vi "LightOffCommand_Create.vi"(8 "error in (no error)":errorcluster, 10 "Light":refnum<class "Light.lvclass">, 11 "reference in":refnum<class "LightOffCommand.lvclass">) -> (0 "error out":errorcluster, 3 "reference out":refnum<class "LightOffCommand.lvclass">)   [LabVIEW 2020, in "LightOffCommand.lvclass"]
uses:
  LightOffCommand.lvclass
  C:/Projects/OpenGDS_DesignPatterns/Command1/Command_class/Command.lvclass
  Light_class/Light.lvclass
  Command_class/Command.lvclass
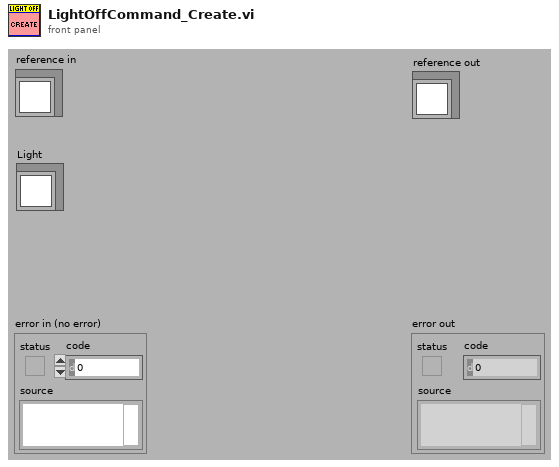
[diagram p1: front panel]
types:
  T1 = typedef "LightOffCommand.lvclass/ObjectAttributes.ctl" = cluster{"Light":refnum<class "Light.lvclass">}
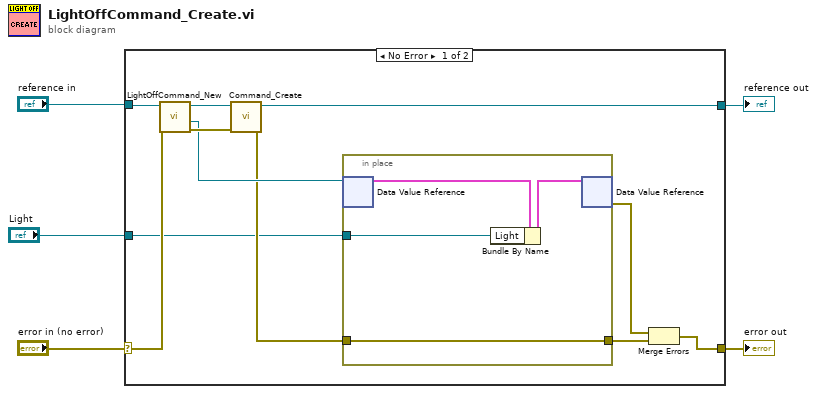
[diagram p0: block diagram]
diagram:
  n1 = case shown="No Error" "error in (no error)" {
    selector: "error in (no error)" -> [w13 w22]
    tunnel: [w11 w22] -> w4
    tunnel: "reference in" -> [w15 w21]
    tunnel: [w10 w21] -> w2
    tunnel: "Light" -> [w6 _]
    frame No Error {
      n2 = call "LightOffCommand_New.vi"("error in (no error)"=w13, "reference in"=w15) -> ("error out"=w14:errorcluster, "DVRRefOut"=w9:refnum<data-value>, "reference out"=w16:refnum<class "LightOffCommand.lvclass">)  [unwired: 6 in, 1 out]
      n3 = call "Command_Create.vi"("error in (no error)"=w14, "reference in"=w16) -> ("error out"=w8:errorcluster, "reference out"=w10:refnum<class "LightOffCommand.lvclass">)  [unwired: 8 in]
      n4 = in-place {
        in-place-border: w8 -> [w18]
        in-place-border: [w18] -> w7
        in-place-border: w6 -> [w17]
        n5 = in-place-dvr #1(w9) -> (w19:T1)  [unwired: 1 out]
        n6 = Bundle By Name(cluster=w19, "Light"=w17) -> (w20:T1)
        n7 = in-place-dvr #1(w20) -> (w12:errorcluster)  [unwired: 1 out]
      }
      n8 = Merge Errors(w12, w7) -> (w11:errorcluster)
    }
    frame Error {
    }
  }
  "error out" <- w4
  "reference out" <- w2
